vi "Coord window-Set column header name.vi"() -> (0 "error out":errorcluster)   [LabVIEW 2020]
uses:
  Globals/Coord window-Globals.vi
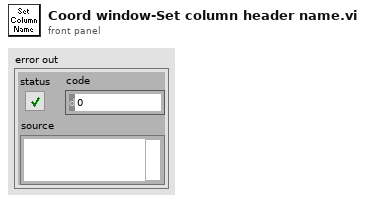
[diagram p1: front panel]
types:
  T1 = typedef "LVRowAndColumnTypeDef.ctl" = cluster{"Row":i32, "Column":i32}
  T2 = typedef "Coordinate list window refs.ctl" = cluster{"Window Name (i.e. Key)":string, "menu reference":refnum<k9>, "VI's reference":refnum<vi>, "Pane 1":refnum<vi>, "Pane 2":refnum<vi>, "Coord Listbox":refnum<vi>, "File name":refnum<vi>, "Picture Map":refnum<vi>, "Stage XYZ Position ind.":refnum<vi>}
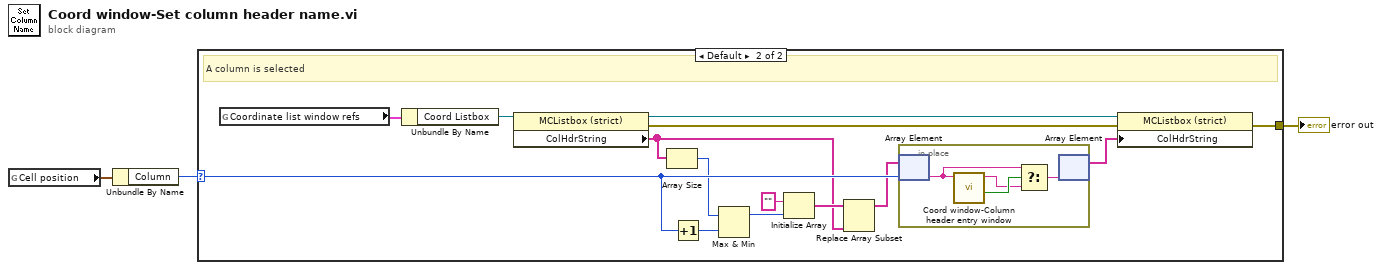
[diagram p0: block diagram]
diagram:
  n1 = global read "Coord window-Globals.vi" "Cell position"() -> (w2:T1)
  n2 = Unbundle By Name(w2) -> ("Column"=w1:i32)
  n3 = case shown="Default" w1 {
    selector: w1 -> [_ w11]
    tunnel: [_ w13] -> w3
    frame -1 {
      # "No column selected! (Fail-safe case)"
    }
    frame Default {
      # "A column is selected"
      n4 = global read "Coord window-Globals.vi" "Coordinate list window refs"() -> (w15:T2)
      n5 = Unbundle By Name(w15) -> ("Coord Listbox"=w16:refnum<vi>)
      n6 = property on="Property Node" class="MCListbox (strict)"(reference=w16) -> (reference out=w17:refnum<vi>, error out=w14:errorcluster, "ColHdrString"=w7:string[])  [unwired: 1 in]
      n7 = Array Size(array=w7) -> (size(s)=w6:i32)
      n8 = Increment(x=w11) -> (x+1=w5:i32)
      n9 = Max & Min(x=w6, y=w5) -> (max(x,y)=w4:i32)  [unwired: 1 out]
      n10 = Initialize Array("", w4) -> (w9:string[])
      n11 = Replace Array Subset(array=w9, new element=w7) -> (w8:string[])  [unwired: 1 in]
      n12 = in-place {
        n13 = in-place-array #1(w8, w11) -> (w20:string)
        n14 = call "Coord window-Column header entry window.vi"("Column name in"=w20) -> ("Cancelled"=w21:bool, "Column name out"=w18:string)  [unwired: 9 in]
        n15 = Select(t=w20, s=w21, f=w18) -> (s? t:f=w19:string)
        n16 = in-place-array #1(w19) -> (w12:string[])  [unwired: 1 out]
      }
      n17 = property on="Property Node" class="MCListbox (strict)"(reference=w17, error in=w14, "ColHdrString"=w12) -> (error out=w13:errorcluster)  [unwired: 1 out]
    }
  }
  "error out" <- w3
